vi "New data getter.vi"(8 "error in":errorcluster, 10 "Child rows":string[][](array[string]), 11 "Root row":string[](array[string])) -> (0 "error in":errorcluster, 3 "Root + child rows":string[][](array[string]))   [LabVIEW 2025, in "CAN-LIN Raw Bus Capture UI.lvlib"]
uses:
  CAN-LIN Raw Bus Capture UI.lvlib
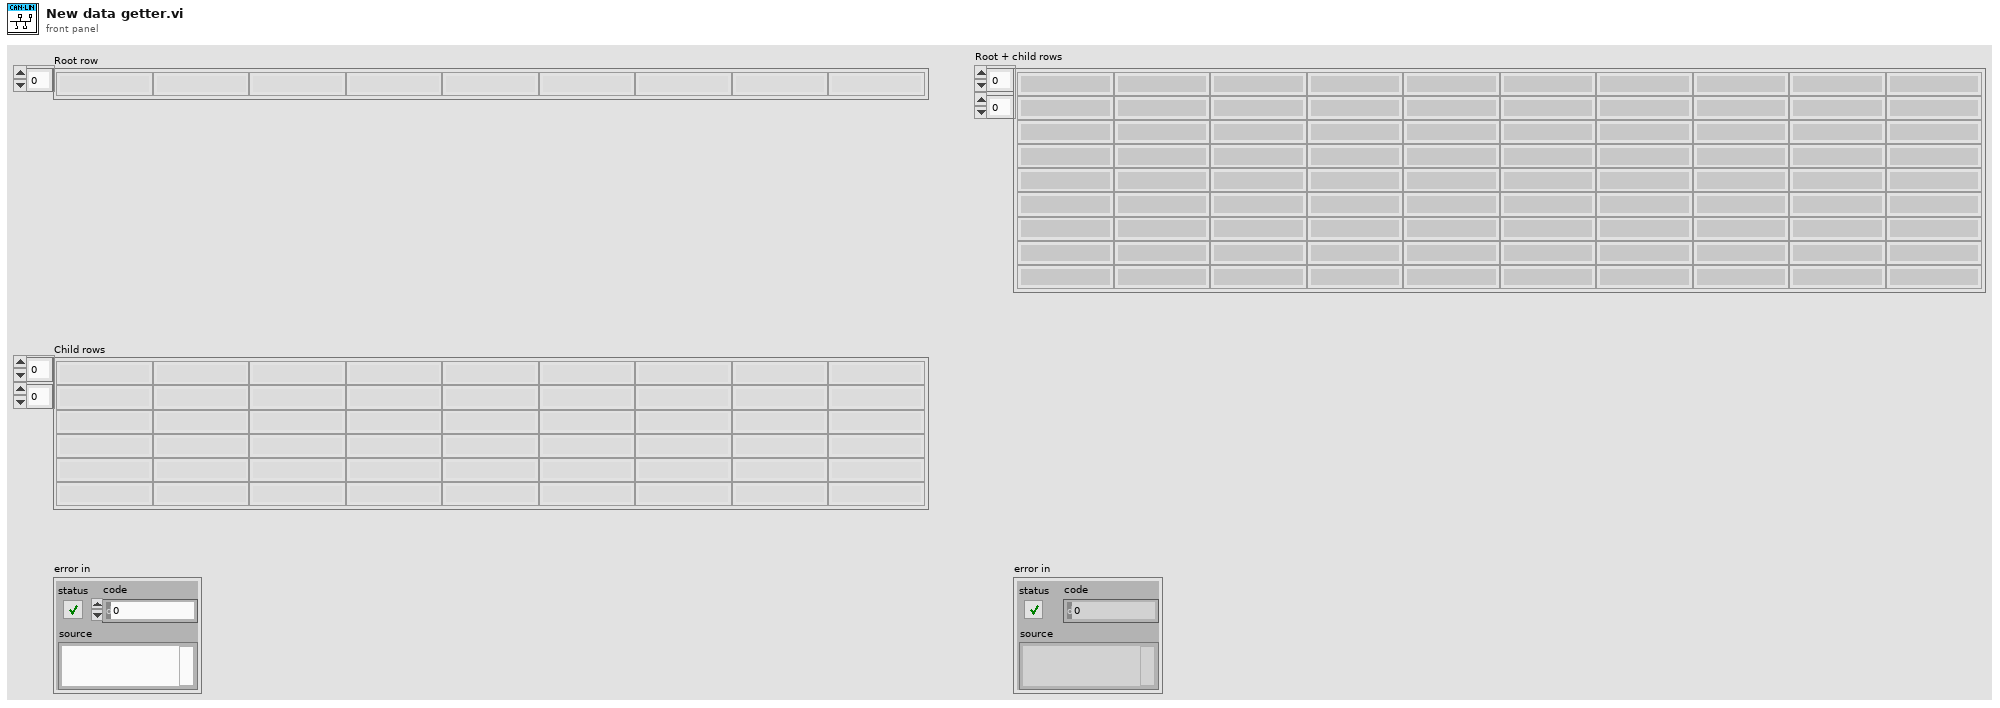
[diagram p1: front panel]
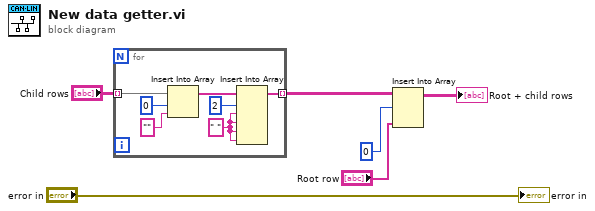
[diagram p0: block diagram]
diagram:
  n1 = for {
    tunnel: "Child rows" -> [w7] mode=indexing
    tunnel: [w11] -> w2 mode=indexing
    w12 = " " ("new element/subarray")
    n2 = Insert Into Array(array=w7, index=0, new element="" ("new element/subarray")) -> (w8:string[])
    n3 = Insert Into Array(array=w8, index=2, new element #1=w12, new element #2=w12, new element #3=w12, new element #4=w12) -> (w11:string[])
  }
  n4 = Insert Into Array(array=w2, index (row)=0, new element="Root row") -> (→"Root + child rows":string[][])  [unwired: 1 in]
  "error in" <- "error in"
